vi "Redisplay SLM.vi"   [LabVIEW 2014]
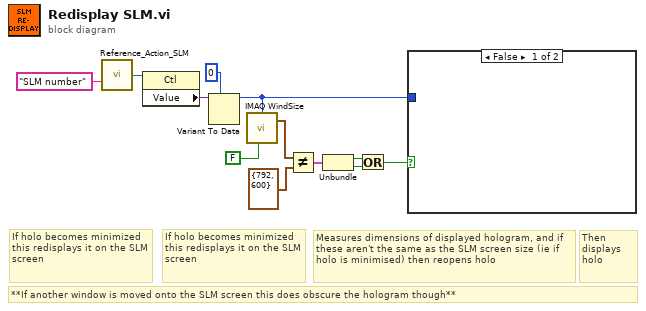
[diagram p0: block diagram]
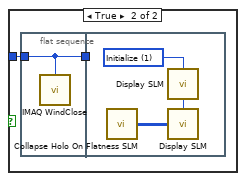
[diagram p2: hidden frame]
diagram:
  # "Then displays holo"
  # "**If another window is moved onto the SLM screen this does obscure the hologram though**"
  # "Measures dimensions of displayed hologram, and if these aren't the same as the SLM screen size (ie if holo is minimised) then reopens holo"
  # "If holo becomes minimized this redisplays it on the SLM screen"
  # "If holo becomes minimized this redisplays it on the SLM screen"
  n1 = call "Reference_Action_SLM.vi"("Control Name"="SLM number") -> ("Ref OUT"=w10:refnum<vi>)  [unwired: 12 in, 2 out]
  n2 = property class="Ctl"(reference=w10) -> ("Value"=w11:variant)  [unwired: 1 in, 2 out]
  n3 = Variant To Data(type=0, Variant=w11) -> (data=w1:i32)  [unwired: 1 in, 1 out]
  n4 = call "IMAQ WindSize"("Get/Set Status? (Set)"=FALSE, "Window Number"=w1) -> ("Width & Height out"=w3:cluster{"Width":i32, "Height":i32})  [unwired: 3 in, 3 out]
  n5 = Not Equal?(x=w3, y=cluster{"Width":i32, "Height":i32} {"Width"=792, "Height"=600} ("Width & Height out 2")) -> (x != y?=w7:cluster{"Width":bool, "Height":bool})
  n6 = Unbundle(w7) -> ("Width"=w6:bool, "Height"=w5:bool)
  n7 = Or(x=w6, y=w5) -> (x .or. y?=w2:bool)
  n8 = case shown="False" w2 {
    tunnel: w1 -> [_ w14]
    frame False {
    }
    frame True {
      n9 = flat-sequence {
        tunnel: w14 -> [w15]
        tunnel: [w15] -> w13
        tunnel: w13 -> [_]
        frame #0 {
          n10 = call "IMAQ WindClose"("Window Number (0...15)"=w15) -> ()  [unwired: 2 in, 4 out]
        }
        frame #1 {
          w18 = u16 1 items=["Read", "Initialize"] ("Action")
          n11 = call "Collapse Holo On Flatness SLM.vi"() -> ("displayed matrix"=w17:u8[][])  [unwired: 15 in]
          n12 = call "Display SLM.vi"("Action"=w18) -> ("Read action"=w16:u16)  [unwired: 14 in]
          n13 = call "Display SLM.vi"("Action"=w16, "displayed matrix"=w17) -> ()  [unwired: 13 in, 1 out]
        }
      }
    }
  }
